vi "Open gRPC Server-Client [2] - Code Generator.vi"   [LabVIEW 2020]
panel:
  # "Open gRPC Server-Client[2] - Code Generator..."
types:
  T1 = enum32{"Invalid", "Standard", "Closed", "Hidden", "Minimized", "Maximized"}
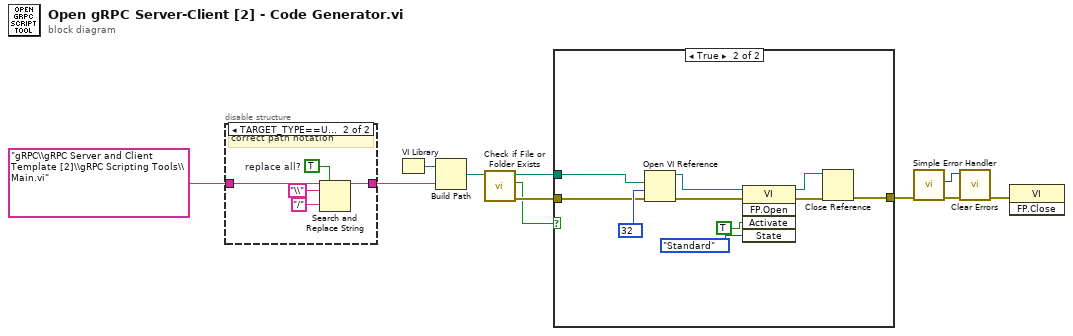
[diagram p0: block diagram]
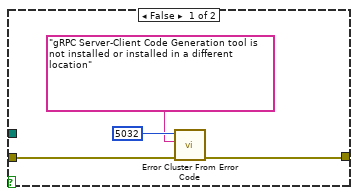
[diagram p3: hidden frame]
diagram:
  n1 = disable-structure shown="TARGET_TYPE==Unix" {
    disable-tunnel: "gRPC\\gRPC Server and Client Template [2]\\gRPC Scripting Tools\\Main.vi" ("name or relative path") -> [w12 w17]
    disable-tunnel: [w12 w16] -> w1
    frame condition #0 {
    }
    frame condition #1 (active) {
      w15 = TRUE  # replace all?
      # "correct path notation"
      n2 = Search and Replace String(replace all?=w15, input string=w17, search string="\\", replace string="/" ("replace string (\"\")")) -> (result string=w16:string)  [unwired: 4 in, 3 out]
    }
  }
  n3 = VI Library() -> (path=w11:path)
  n4 = Build Path(base path=w11, name or relative path=w1) -> (appended path=w10:path)
  n5 = call <vilib>:"Check if File or Folder Exists.vi"("path"=w10) -> ("error out"=w9:errorcluster, "file or folder exists?"=w7:bool, "dup path"=w8:path)  [unwired: 8 in]
  n6 = case shown="True" w7 {
    tunnel: w9 -> [w21 w30]
    tunnel: w8 -> [_ w29]
    tunnel: [w20 w22] -> w6
    frame False {
      n7 = call <vilib>:"Error Cluster From Error Code.vi"("error in (no error)"=w21, "error message (\"\")"="gRPC Server-Client Code Generation tool is not installed or installed in a different location" ("error message (\"\")"), "error code (0)"=5032) -> ("error out"=w20:errorcluster)  [unwired: 6 in]
    }
    frame True {
      n8 = Open VI Reference(vi path=w29, options=32, error in (no error)=w30) -> (vi reference=w28:refnum<vi>, error out=w27:errorcluster)  [unwired: 3 in]
      n9 = invoke class="VI" method="FP.Open"(reference=w28, error in=w27, "Activate"=TRUE ("Activate?"), "State"=T1."Standard") -> (reference out=w23:refnum<vi>, error out=w24:errorcluster)  [unwired: 1 in, 3 out]
      n10 = Close Reference(reference=w23, error in (no error)=w24) -> (error out=w22:errorcluster)
    }
  }
  n11 = call <vilib>:"Simple Error Handler.vi"("error in (no error)"=w6) -> ("code out"=w4:i32, "error out"=w5:errorcluster)  [unwired: 4 in, 3 out]
  n12 = call <vilib>:"Clear Errors.vi"("error in (no error)"=w5, "specific error code to clear (0: all)"=w4) -> ("error out"=w3:errorcluster)  [unwired: 4 in, 1 out]
  n13 = invoke class="VI" method="FP.Close"(error in=w3) -> ()  [unwired: 2 in, 3 out]
